vi "Channel Registration.vi"() -> ()   [LabVIEW 2021]
uses:
  Hardware Configuration/Hardware Configuration Controls/Device Type.ctl
  Hardware Configuration/Hardware Configuration Controls/Device Function.ctl
  <vilib>/vision/Image Controls.llb/IMAQ Image.ctl
  Channel Reg Controls/Channel Reg Notifier Type.ctl
  Channel Reg Controls/Channel Reg Actions.ctl
  Device Library/Cameras/Hamamatsu/Orca Flash/Orca Flash Controls/Orca Flash Actions.ctl
  Device Library/Stages/Stages Controls/Stage Actions.ctl
  Channel Reg Sub VI/Reg Counter Action.ctl
  Device Library/Cameras/Camera Controls/Camera IMAQ Key Info.ctl
  <vilib>/vision/NI_Vision_Development_Module.lvlib
panel:
  in  "Edge Size":i32
  in  "Base Save Path":path
  in  "Save Name":string
  in  "Subfolder Name":string="Area"
  in  "Quit":bool
  in  "No. of Steps":i32
  in  "Start Register":bool
  out "Bead Y Pos (µm)":dbl
  out "Bead X Pos (µm)":dbl
  in  "Move To Corner":bool
  in  "Pixel Size (µm)":dbl
  in  "Get Bead":bool
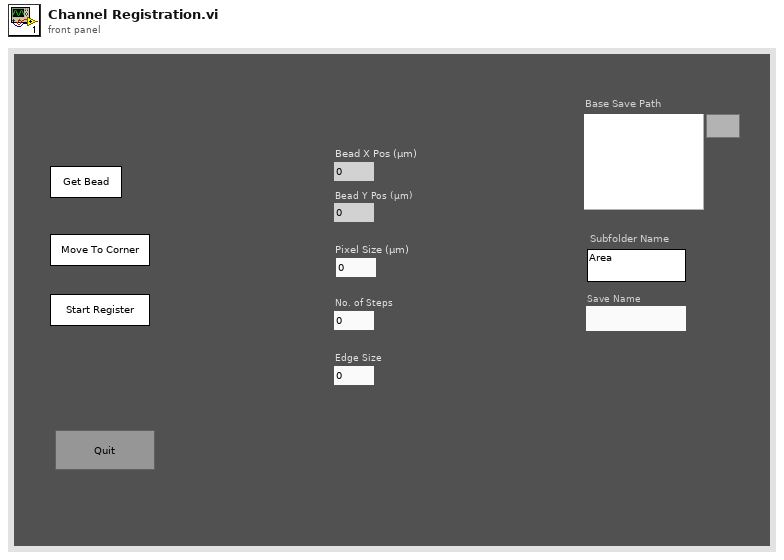
[diagram p1: front panel]
types:
  T1 = typedef "Orca Flash Actions.ctl" = enum16{"IDLE", "PREVIEW", "RECORD", "Send Trigger", "SOFT TRIGGER", "Record Settings", "SETPARAM", "GETPARAM", "SETROI", "GETROI", "PROGRESSIVE MODE", "AREA MODE", "STATUS", "QUIT"}
  T2 = typedef "Channel Reg Notifier Type.ctl" = cluster{"Action":T3, "Display Image":T4, "Init X Pos":dbl, "Init Y Pos":dbl, "Quads":T4[], "Add Quads":T4[], "Camera Image":T4, "Camera Notifier Name":string, "Stage Notifier Name":string, "X Grid Pos":dbl[], "Y Grid Pos":dbl[], "Pixel Size":dbl, "No. of Steps":i32, "Edge Size":i32, "Relative X":dbl, "Relative Y":dbl, "Scan Done?":bool}
  T3 = typedef "Channel Reg Actions.ctl" = enum16{"Start Register", "Get Bead", "Move To Corner", "Get Quad", "Add Quad", "Move Stage", "Save Image", "Exit", "Quit"}
  T4 = typedef "IMAQ Image.ctl" = refnum<image>
  T5 = typedef "Device Function.ctl" = enum16{"Primary", "Secondary", "Overview", "Wide Field Drift Correction", "642 nm Excitation", "560 nm Excitation", "940 nm Excitation", "546 nm Excitation", "488 nm Excitation", "405 nm Excitation", "Objective Drift Correction", "4Pi Focus Lock", "4Pi Objective Lock", "Objective XY", "Objective Z", "Sample XY", "Sample Coarse Z", "Sample Z", "4Pi Lower", "4Pi Upper", "Em Small", "Em Large", "Ex Small", "Ex Large", "Mojo", "Adj Cavity", "Line Scanning", "Alert"}
  T6 = typedef "Device Type.ctl" = enum16{"AOTF", "Camera", "Deformable Mirror", "Laser", "Flip Mirror", "Shutter", "Stage", "Waveform", "FPGA", "Email"}
  T7 = typedef "Image Type" = u32
  T8 = typedef "Stage Actions.ctl" = enum16{"Get Position", "SERVO OFF", "SERVO ON", "SERVO ON/OFF", "MVR", "MOVE", "HALT", "ONTARGET", "ERROR", "REFERENCE", "INIT", "VELOCITY", "STATUS", "EXIT", "HOME", "ZEROPOS", "NANOPOS", "ANALOG", "QUIT"}
  T9 = typedef "Reg Counter Action.ctl" = enum16{"Initialize", "Update Count"}
  T10 = typedef "Camera IMAQ Key Info.ctl" = cluster{"Frame":u32, "Sensor Height":i32, "Sensor Width":i32, "ROI Height":i32, "ROI Width":i32, "ROI Enable?":bool, "Bit per Pixel":u8}
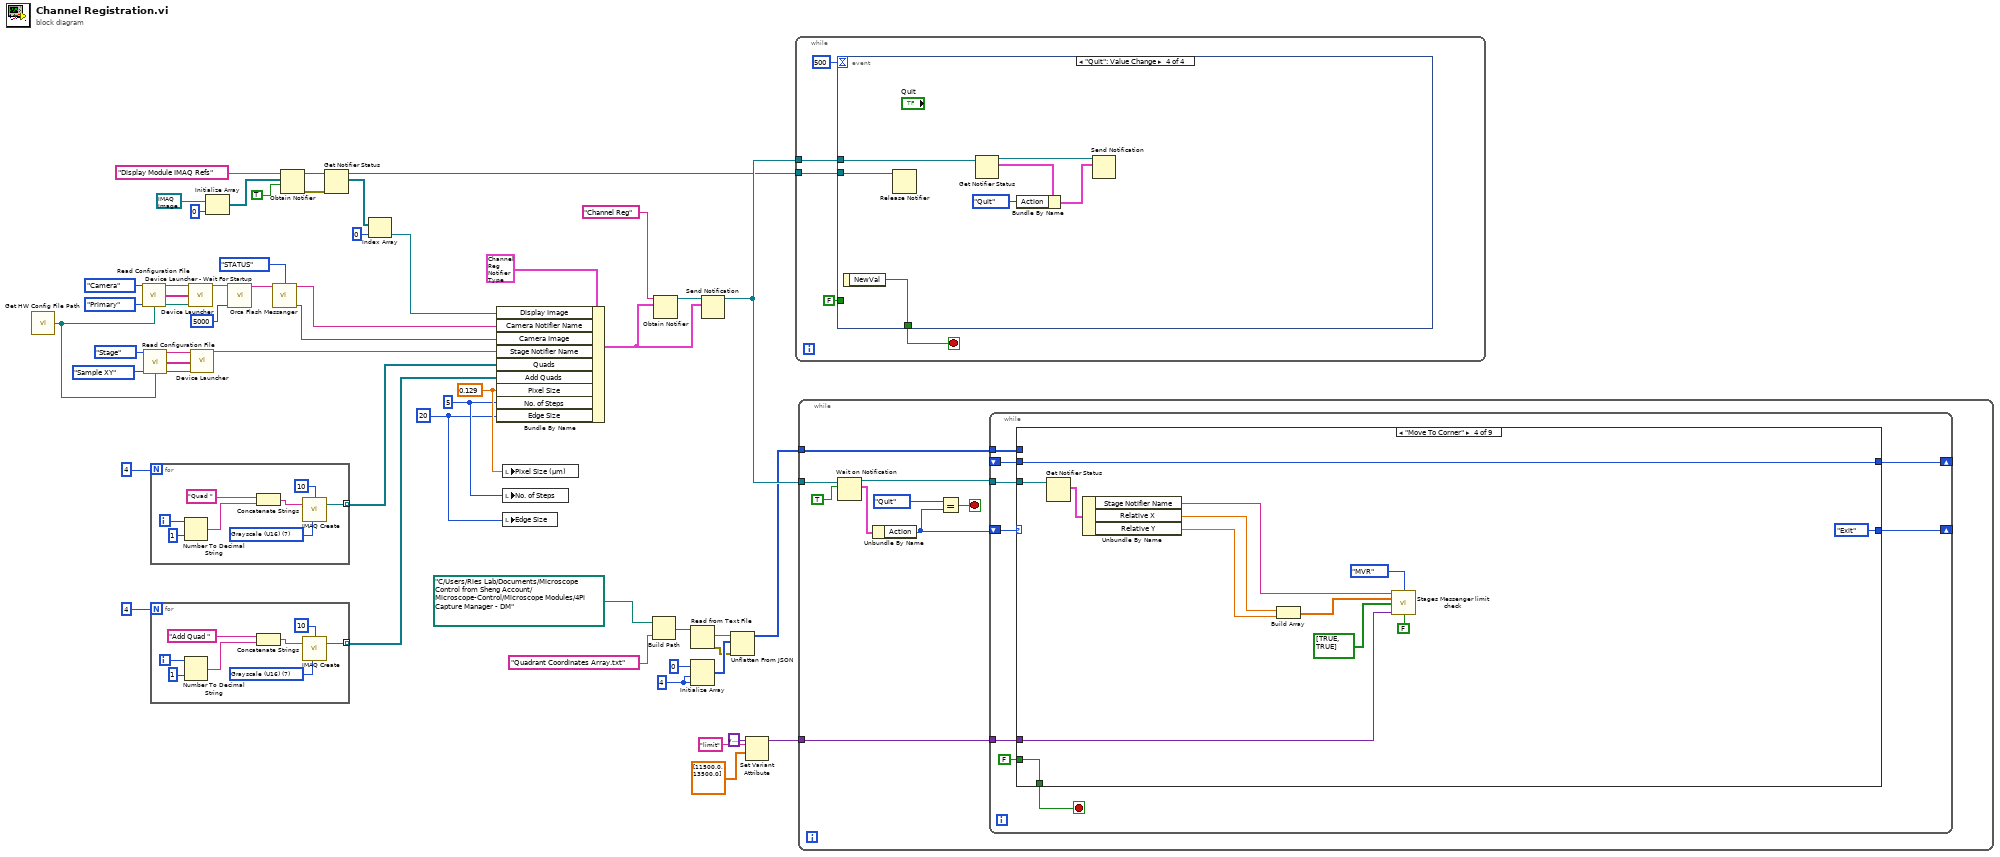
[diagram p0: block diagram]
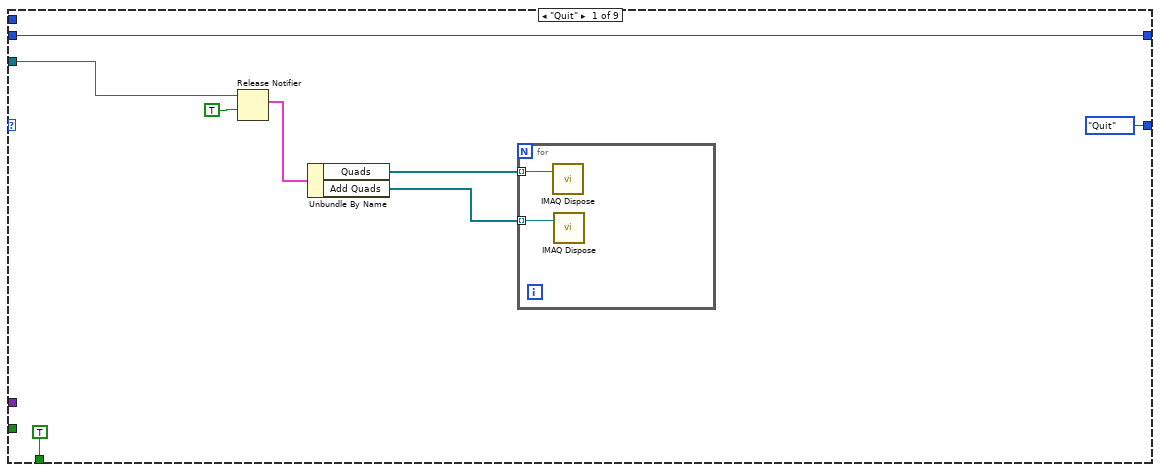
[diagram p2: hidden frame]
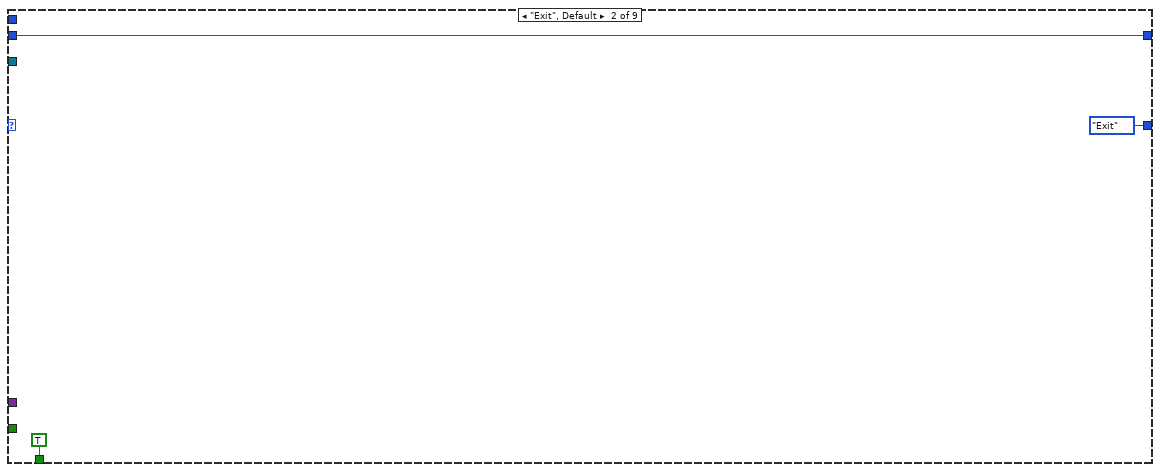
[diagram p3: hidden frame]
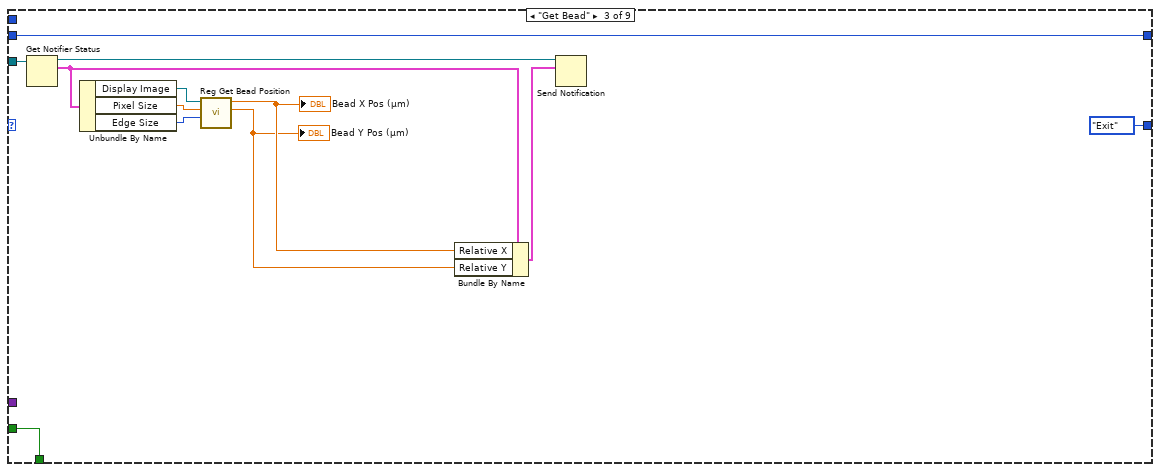
[diagram p4: hidden frame]
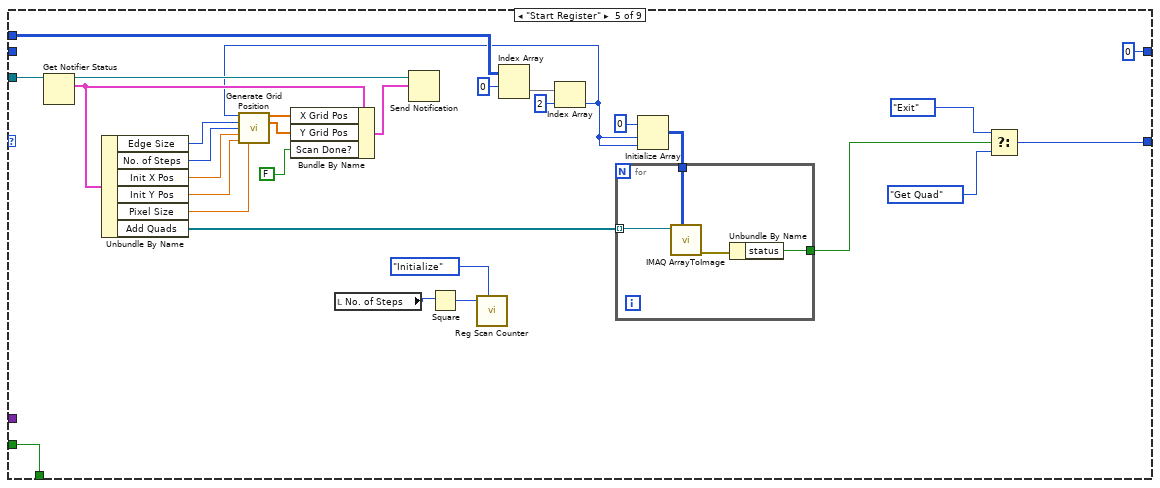
[diagram p5: hidden frame]
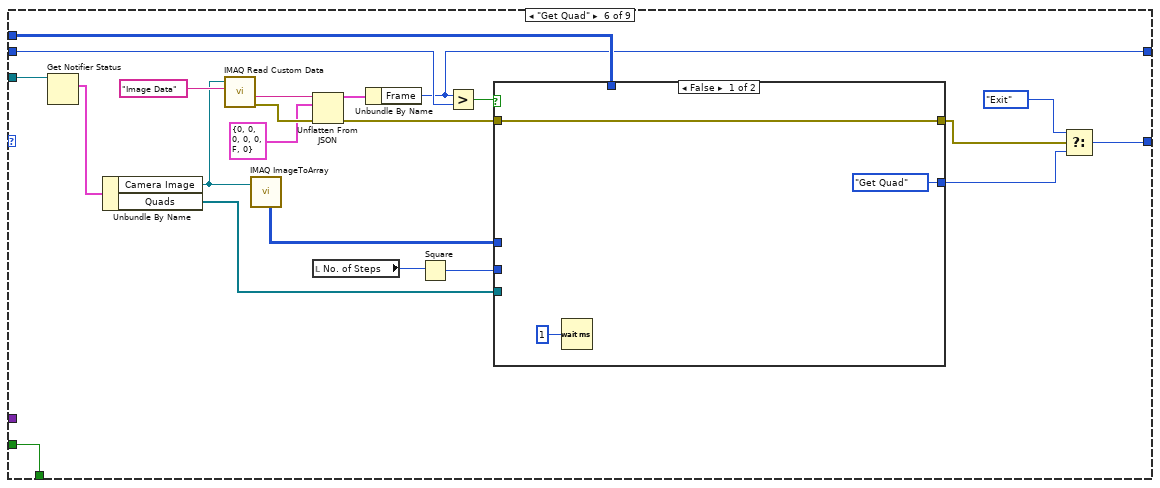
[diagram p6: hidden frame]
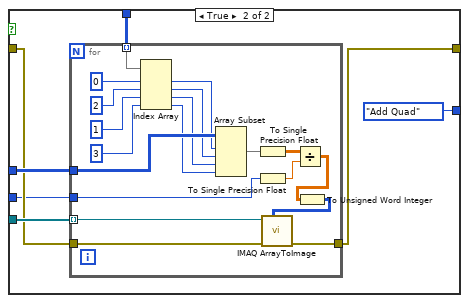
[diagram p7: hidden frame]
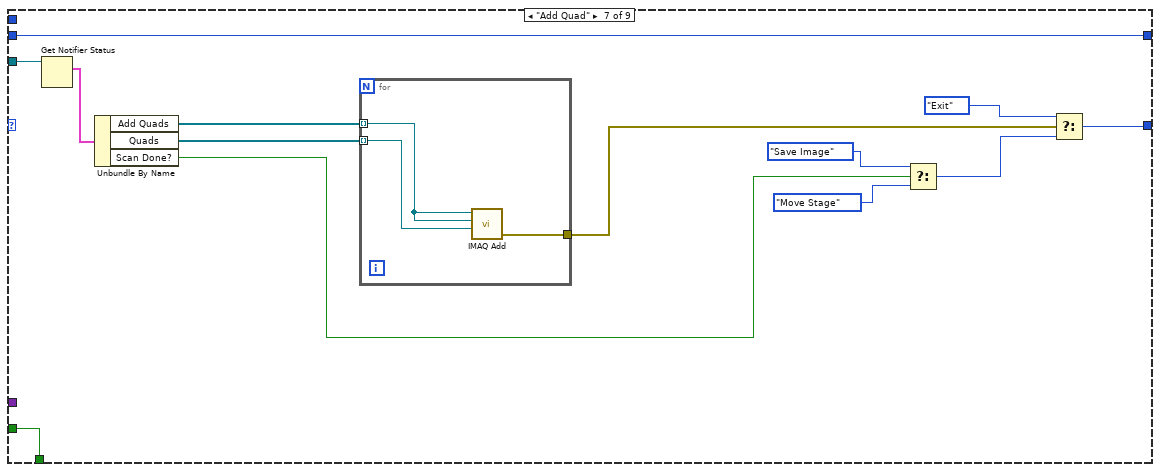
[diagram p8: hidden frame]
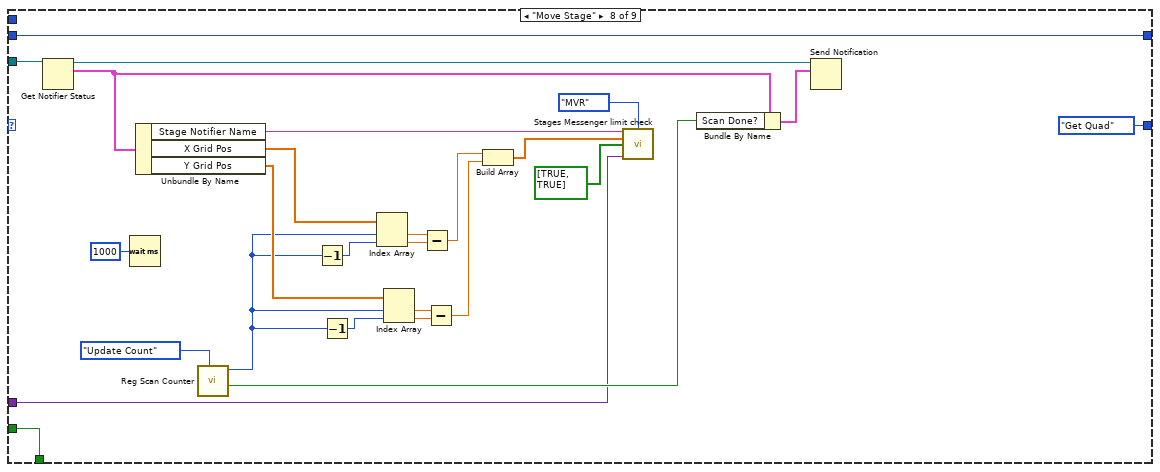
[diagram p9: hidden frame]
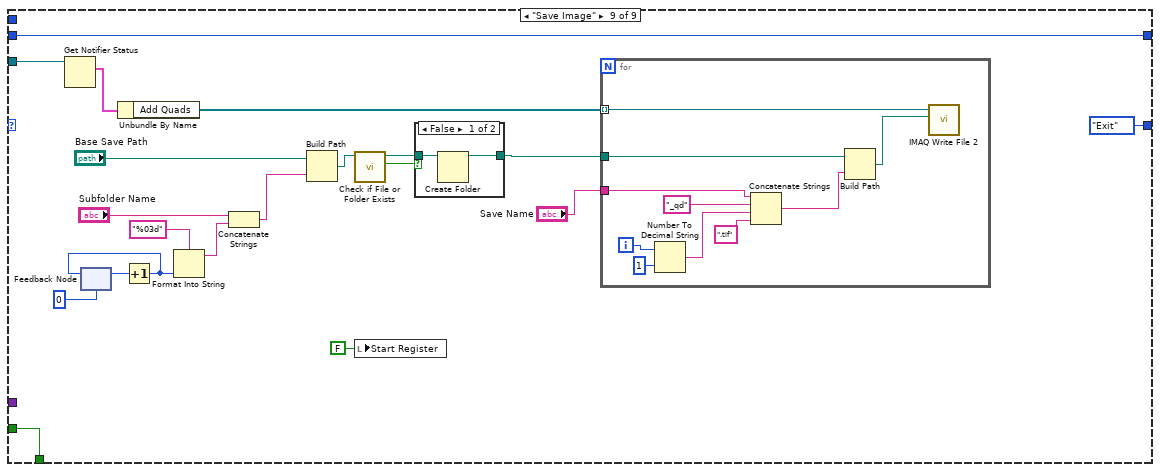
[diagram p10: hidden frame]
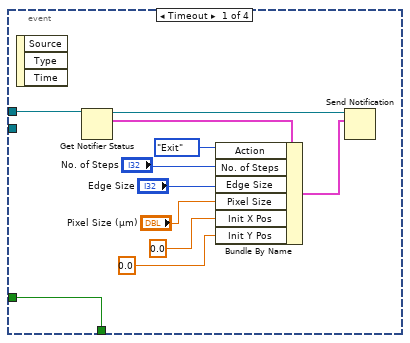
[diagram p12: hidden frame]
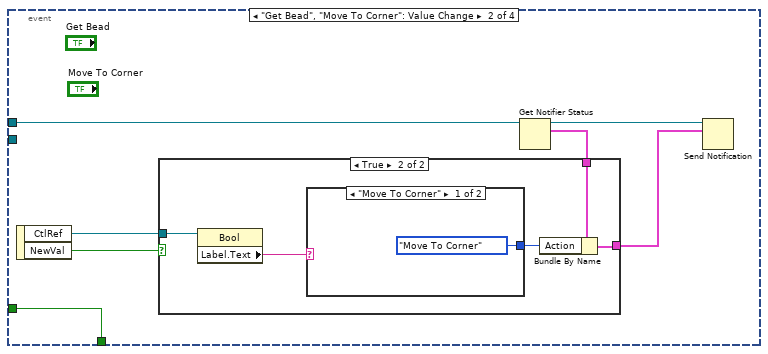
[diagram p13: hidden frame]
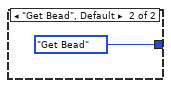
[diagram p15: hidden frame]
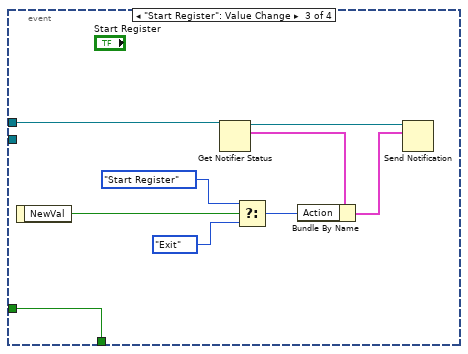
[diagram p16: hidden frame]
diagram:
  w1 = 20 ("Edge Size")
  w2 = 5 ("No. of Steps")
  w3 = 0.129 ("Pixel Size")
  w18 = 4 ("dimension size")
  n1 = call "Get HW Config File Path.vi"() -> ("File Path"=w49:path)  [unwired: 14 in, 1 out]
  n2 = call "Read Configuration File.vi"("Device Type"=Device_Type."Camera", "Device Function"=Device_Function."Primary", "Config File Path"=w49) -> ("Unique Notifier Name"=w50:string, "Device Ports/IDs/Channels"=w52:string[], "Device Engine Path"=w51:path)  [unwired: 9 in, 1 out]
  n3 = call "Read Configuration File.vi"("Device Type"=Device_Type."Stage", "Device Function"=Device_Function."Sample XY", "Config File Path"=w49) -> ("Unique Notifier Name"=w46:string, "Device Ports/IDs/Channels"=w45:string[], "Device Engine Path"=w44:path)  [unwired: 9 in, 1 out]
  n4 = for {
    N: 4 -> [_]
    tunnel: [w60] -> w27 mode=indexing
    i -> [w59]
    w62 = T7 7 items=["Grayscale (U8)", "Grayscale (I16)", "Grayscale (SGL)", "Complex (CSG)", "RGB (U32)", "HSL (U32)", "RGB (U64)", "Grayscale (U16)"] ("Image Type")
    n5 = Number To Decimal String(number=w59, width (-)=i16 1) -> (decimal integer string=w56:string)
    n6 = Concatenate Strings("Quad " ("Image Name"), w56) -> (w55:string)
    n7 = call "IMAQ Create"("Border Size"=10, "Image Name"=w55, "Image Type"=w62) -> ("New Image"=w60:T4)  [unwired: 2 in, 1 out]
  }
  n8 = for {
    N: 4 -> [_]
    tunnel: [w68] -> w25 mode=indexing
    i -> [w67]
    w70 = T7 7 items=["Grayscale (U8)", "Grayscale (I16)", "Grayscale (SGL)", "Complex (CSG)", "RGB (U32)", "HSL (U32)", "RGB (U64)", "Grayscale (U16)"] ("Image Type")
    n9 = Number To Decimal String(number=w67, width (-)=i16 1) -> (decimal integer string=w64:string)
    n10 = Concatenate Strings("Add Quad " ("Image Name"), w64) -> (w63:string)
    n11 = call "IMAQ Create"("Border Size"=10, "Image Name"=w63, "Image Type"=w70) -> ("New Image"=w68:T4)  [unwired: 2 in, 1 out]
  }
  n12 = call "Device Launcher.vi"("Notifier Name"=w50, "Device Ports/IDs/Channels"=w52, "Device Engine Path"=w51) -> ("Notifier Name"=w16:string)  [unwired: 11 in, 1 out]
  n13 = call "Device Launcher.vi"("Notifier Name"=w46, "Device Ports/IDs/Channels"=w45, "Device Engine Path"=w44) -> ("Notifier Name"=w10:string)  [unwired: 11 in, 1 out]
  n14 = Initialize Array(T4 refnum ("New Image"), 0 ("dimension size")) -> (w39:T4[])
  n15 = call "Device Launcher - Wait For Startup.vi"("Notifier Name"=w16, "Wait Time (ms)"=5000) -> ("Notifier Name (Dup)"=w14:string)  [unwired: 12 in, 1 out]
  n16 = call "Orca Flash Messanger.vi"("Notifier Name"=w14, "Camera Actions"=Orca_Flash_Actions."STATUS") -> ("Notifier Name Dup"=w11:string, "Image Ref"=w12:T4)  [unwired: 9 in, 3 out]
  n17 = Obtain Notifier(name (unnamed)="Display Module IMAQ Refs", notification data type=w39, create if not found? (T)=TRUE) -> (notifier out=w38:refnum<notifier>, error out=w37:errorcluster)  [unwired: 1 in, 1 out]
  n18 = Get Notifier Status(notifier=w38, error in (no error)=w37) -> (notifier out=w9:refnum<notifier>, current notification=w36:T4[])  [unwired: 3 out]
  n19 = Index Array(array=w36, index=0) -> (element=w33:T4)
  n20 = Bundle By Name(cluster=T2 {"Action"=enum."Get Bead", "Display Image"=refnum, "Init X Pos"=0.0, "Init Y Pos"=0.0, "Quads"=[], "Add Quads"=[], "Camera Image"=refnum, "Camera Notifier Name"="", "Stage Notifier Name"="", "X Grid Pos"=[], "Y Grid Pos"=[], "Pixel Size"=0.0, "No. of Steps"=0, "Edge Size"=0, "Relative X"=0.0, "Relative Y"=0.0, "Scan Done?"=FALSE} ("Channel Reg Notifier Type"), "Display Image"=w33, "Camera Notifier Name"=w11, "Camera Image"=w12, "Stage Notifier Name"=w10, "Quads"=w27, "Add Quads"=w25, "Pixel Size"=w3, "No. of Steps"=w2, "Edge Size"=w1) -> (w30:T2)
  n21 = local write "Pixel Size (µm)"(w3) -> ()
  n22 = local write "No. of Steps"(w2) -> ()
  n23 = local write "Edge Size"(w1) -> ()
  n24 = Build Path(base path=path "C:/Users/Ries Lab/Documents/Microscope Control from Sheng Account/Microscope-Control/Microscope Modules/4Pi Capture Manager - DM" ("path"), name or relative path="Quadrant Coordinates Array.txt") -> (appended path=w21:path)
  n25 = Obtain Notifier(name (unnamed)="Channel Reg", notification data type=w30) -> (notifier out=w31:refnum<notifier>)  [unwired: 2 in, 2 out]
  n26 = Read from Text File(file (use dialog)=w21) -> (text=w20:string, error out=w19:errorcluster)  [unwired: 3 in, 2 out]
  n27 = Initialize Array(0 ("element"), w18, w18) -> (w22:i32[][])
  n28 = Send Notification(notification=w30, notifier=w31) -> (notifier out=w29:refnum<notifier>)  [unwired: 1 in, 1 out]
  n29 = Unflatten From JSON(JSON string=w20, type and defaults=w22, error in (no error)=w19) -> (value=w17:i32[][])  [unwired: 4 in, 1 out]
  n30 = Set Variant Attribute(Variant=variant ("variant"), name="limit", value=dbl[] [11500.0, 13500.0] ("Array")) -> (Variant out=w5:variant)  [unwired: 1 in, 2 out]
  n31 = while {
    tunnel: w29 -> [w75]
    tunnel: w9 -> [w72]
    stop <- w74 stop-if-true
    n32 = event shown="[3] \"Quit\": Value Change" {
      selector: _ -> [_ _ _ _]
      dyn-events: _ -> [_ _ _ _]
      timeout: 500 -> [_ _ _ _]
      tunnel: w75 -> [w85 w93 w110 w116]
      tunnel: [w86 w87 w102 w117] -> w74
      tunnel: FALSE ("NewVal") -> [w86 w87 w102 _]
      tunnel: w72 -> [_ _ _ w111]
      event Timeout {
        n33 = event-data() -> ()  [unwired: 1 in, 3 out]
        n34 = Get Notifier Status(notifier=w85) -> (notifier out=w78:refnum<notifier>, current notification=w84:T2)  [unwired: 1 in, 3 out]
        n35 = Bundle By Name(cluster=w84, "Action"=Channel_Reg_Actions."Exit", "No. of Steps"="No. of Steps", "Edge Size"="Edge Size", "Pixel Size"="Pixel Size (µm)", "Init X Pos"=0.0, "Init Y Pos"=0.0) -> (w77:T2)
        n36 = Send Notification(notification=w77, notifier=w78) -> ()  [unwired: 1 in, 2 out]
      }
      event "Get Bead", "Move To Corner": Value Change {
        n37 = event-data() -> ("CtlRef"=w88:refnum<vi>, "NewVal"=w89:bool)  [unwired: 1 in]
        n38 = Get Notifier Status(notifier=w93) -> (notifier out=w91:refnum<notifier>, current notification=w92:T2)  [unwired: 1 in, 3 out]
        n39 = case shown="True" w89 {
          tunnel: w92 -> [w94 w99]
          tunnel: [w94 w97] -> w90
          tunnel: w88 -> [_ w96]
          frame False {
          }
          frame True {
            n40 = property class="Bool"(reference=w96) -> ("Label.Text"=w95:string)  [unwired: 1 in, 2 out]
            n41 = case shown="\"Move To Corner\"" w95 {
              tunnel: [Channel_Reg_Actions."Move To Corner" ("Action") Channel_Reg_Actions."Get Bead" ("Action")] -> w98
              frame "Move To Corner" {
              }
              frame "Get Bead", Default {
              }
            }
            n42 = Bundle By Name(cluster=w99, "Action"=w98) -> (w97:T2)
          }
        }
        n43 = Send Notification(notification=w90, notifier=w91) -> ()  [unwired: 1 in, 2 out]
      }
      event "Start Register": Value Change {
        n44 = event-data() -> ("NewVal"=w108:bool)  [unwired: 1 in]
        n45 = Get Notifier Status(notifier=w110) -> (notifier out=w104:refnum<notifier>, current notification=w109:T2)  [unwired: 1 in, 3 out]
        n46 = Select(t=Channel_Reg_Actions."Start Register" ("x"), s=w108, f=Channel_Reg_Actions."Exit") -> (s? t:f=w105:T3)
        n47 = Bundle By Name(cluster=w109, "Action"=w105) -> (w103:T2)
        n48 = Send Notification(notification=w103, notifier=w104) -> ()  [unwired: 1 in, 2 out]
      }
      event "Quit": Value Change {
        n49 = event-data() -> ("NewVal"=w117:bool)  [unwired: 1 in]
        n50 = Release Notifier(notifier=w111) -> ()  [unwired: 2 in, 3 out]
        n51 = Get Notifier Status(notifier=w116) -> (notifier out=w115:refnum<notifier>, current notification=w114:T2)  [unwired: 1 in, 3 out]
        n52 = Bundle By Name(cluster=w114, "Action"=Channel_Reg_Actions."Quit") -> (w113:T2)
        n53 = Send Notification(notification=w113, notifier=w115) -> ()  [unwired: 1 in, 2 out]
      }
    }
  }
  n54 = while {
    tunnel: w29 -> [w126]
    tunnel: w17 -> [w119]
    tunnel: w5 -> [w118]
    stop <- w120 stop-if-true
    n55 = Wait on Notification(notifier=w126, ignore previous (F)=TRUE) -> (notifier out=w123:refnum<notifier>, notification=w124:T2)  [unwired: 2 in, 2 out]
    n56 = Unbundle By Name(w124) -> ("Action"=w122:T3)
    n57 = Equal?(x=Channel_Reg_Actions."Quit", y=w122) -> (x = y?=w120:bool)
    n58 = while {
      tunnel: w123 -> [w135]
      tunnel: w119 -> [w133]
      shift-right: [w132] -> _
      shift-left: w122 -> [w134]
      shift-right: [w130] -> _
      shift-left: _ -> [w131]
      tunnel: w118 -> [w127]
      stop <- w129 stop-if-true
      n59 = case shown="\"Move To Corner\"" w134 {
        tunnel: w135 -> [w143 _ w160 w169 w202 w228 w270 w299 w319]
        tunnel: w133 -> [_ _ _ _ w198 w219 _ _ _]
        tunnel: [Channel_Reg_Actions."Quit" ("f") Channel_Reg_Actions."Exit" ("f") Channel_Reg_Actions."Exit" ("f") Channel_Reg_Actions."Exit" ("f") w191 w212 w263 Channel_Reg_Actions."Get Quad" ("f") Channel_Reg_Actions."Exit" ("f")] -> w132
        tunnel: w131 -> [w142 w148 w155 w167 _ w221 w269 w293 w303]
        tunnel: [w142 w148 w155 w167 u32 0 ("Frame") w210 w269 w293 w303] -> w130
        tunnel: [TRUE TRUE w153 w165 w186 w209 w262 w292 w301] -> w129
        tunnel: FALSE -> [_ _ w153 w165 w186 w209 w262 w292 w301]
        tunnel: w127 -> [_ _ _ w161 _ _ _ w274 _]
        frame "Quit" {
          n60 = Release Notifier(notifier=w143, force destroy? (F)=TRUE) -> (last notification=w140:T2)  [unwired: 1 in, 2 out]
          n61 = Unbundle By Name(w140) -> ("Quads"=w137:T4[], "Add Quads"=w136:T4[])
          n62 = for {
            tunnel: w137 -> [w145] mode=indexing
            tunnel: w136 -> [w144] mode=indexing
            n63 = call "IMAQ Dispose"("Image"=w145) -> ()  [unwired: 5 in, 1 out]
            n64 = call "IMAQ Dispose"("Image"=w144) -> ()  [unwired: 5 in, 1 out]
          }
        }
        frame "Exit", Default {
        }
        frame "Get Bead" {
          n65 = Get Notifier Status(notifier=w160) -> (notifier out=w158:refnum<notifier>, current notification=w157:T2)  [unwired: 1 in, 3 out]
          n66 = Unbundle By Name(w157) -> ("Display Image"=w159:T4, "Pixel Size"=w150:dbl, "Edge Size"=w149:i32)
          n67 = call "Reg Get Bead Position.vi"("Edge size"=w149, "Pixel Size (µm)"=w150, "Image Ref"=w159) -> ("Y Pos"=w151:dbl, "X Pos"=w152:dbl)  [unwired: 7 in]
          "Bead X Pos (µm)" <- w152
          "Bead Y Pos (µm)" <- w151
          n68 = Bundle By Name(cluster=w157, "Relative X"=w152, "Relative Y"=w151) -> (w156:T2)
          n69 = Send Notification(notification=w156, notifier=w158) -> ()  [unwired: 1 in, 2 out]
        }
        frame "Move To Corner" {
          n70 = Get Notifier Status(notifier=w169) -> (current notification=w162:T2)  [unwired: 1 in, 4 out]
          n71 = Unbundle By Name(w162) -> ("Stage Notifier Name"=w168:string, "Relative X"=w163:dbl, "Relative Y"=w164:dbl)
          n72 = Build Array(w163, w164) -> (w171:dbl[])
          n73 = call "Stages Messenger limit check.vi"("Stage Notifier Name"=w168, "Actions"=Stage_Actions."MVR", "Setpoint"=w171, "Axis"=bool[] [TRUE, TRUE], "Misc"=w161, "Exit While Busy?"=FALSE) -> ()  [unwired: 6 in, 4 out]
        }
        frame "Start Register" {
          n74 = Get Notifier Status(notifier=w202) -> (notifier out=w185:refnum<notifier>, current notification=w188:T2)  [unwired: 1 in, 3 out]
          n75 = Unbundle By Name(w188) -> ("Edge Size"=w182:i32, "No. of Steps"=w183:i32, "Init X Pos"=w178:dbl, "Init Y Pos"=w177:dbl, "Pixel Size"=w184:dbl, "Add Quads"=w195:T4[])
          n76 = local read "No. of Steps"() -> (w175:i32)
          n77 = Square(x=w175) -> (x^2=w176:i32)
          n78 = call "Reg Scan Counter.vi"("Action"=Reg_Counter_Action."Initialize", "# of Steps"=w176) -> ()  [unwired: 8 in, 2 out]
          n79 = Index Array(array=w198, index (row)=0) -> (element=w200:i32[])  [unwired: 1 in]
          n80 = Index Array(array=w200, index=2) -> (element=w181:i32)
          n81 = call "Generate Grid Position.vi"("Image Size"=w181, "Edge Size"=w182, "# of Steps"=w183, "init x pos"=w178, "init y pos"=w177, "Pixel Size"=w184) -> ("x grid pos"=w180:dbl[], "y grid pos"=w179:dbl[])  [unwired: 8 in]
          n82 = Bundle By Name(cluster=w188, "X Grid Pos"=w180, "Y Grid Pos"=w179, "Scan Done?"=FALSE) -> (w187:T2)
          n83 = Send Notification(notification=w187, notifier=w185) -> ()  [unwired: 1 in, 2 out]
          n84 = Initialize Array(u16 0 ("index"), w181, w181) -> (w196:u16[][])
          n85 = for {
            tunnel: w196 -> [w206]
            tunnel: w195 -> [w205] mode=indexing
            tunnel: [w203] -> w194
            n86 = call "IMAQ ArrayToImage"("Image Pixels (U16)"=w206, "Image"=w205) -> ("error out"=w204:errorcluster)  [unwired: 8 in, 1 out]
            n87 = Unbundle By Name(w204) -> ("status"=w203:bool)
          }
          n88 = Select(t=Channel_Reg_Actions."Exit" ("x"), s=w194, f=Channel_Reg_Actions."Get Quad") -> (s? t:f=w191:T3)
        }
        frame "Get Quad" {
          n89 = Get Notifier Status(notifier=w228) -> (current notification=w227:T2)  [unwired: 1 in, 4 out]
          n90 = Unbundle By Name(w227) -> ("Camera Image"=w218:T4, "Quads"=w216:T4[])
          n91 = call "IMAQ Read Custom Data"("Key"="Image Data", "Image"=w218) -> ("error out"=w226:errorcluster, "Custom Data Out"=w225:string)  [unwired: 7 in, 1 out]
          n92 = call "IMAQ ImageToArray"("Image"=w218) -> ("Image Pixels (U16)"=w217:u16[][])  [unwired: 3 in, 4 out]
          n93 = Unflatten From JSON(JSON string=w225, type and defaults=T10 {"Frame"=0, "Sensor Height"=0, "Sensor Width"=0, "ROI Height"=0, "ROI Width"=0, "ROI Enable?"=FALSE, "Bit per Pixel"=0} ("Camera IMAQ Key Info"), error in (no error)=w226) -> (value=w223:T10, error out=w215:errorcluster)  [unwired: 4 in]
          n94 = local read "No. of Steps"() -> (w208:i32)
          n95 = Unbundle By Name(w223) -> ("Frame"=w210:u32)
          n96 = Square(x=w208) -> (x^2=w207:i32)
          n97 = Greater?(x=w210, y=w221) -> (0:w220:bool)
          n98 = case shown="False" w220 {
            tunnel: w216 -> [_ w238]
            tunnel: w219 -> [_ w237]
            tunnel: w217 -> [_ w236]
            tunnel: w215 -> [w230 w235]
            tunnel: [w230 w234] -> w214
            tunnel: [Channel_Reg_Actions."Get Quad" ("f") Channel_Reg_Actions."Add Quad" ("f")] -> w211
            tunnel: w207 -> [_ w232]
            frame False {
              n99 = Wait (ms)(milliseconds to wait=u32 1) -> ()  [unwired: 1 out]
            }
            frame True {
              n100 = for {
                tunnel: w238 -> [w256] mode=indexing
                tunnel: w236 -> [w257]
                tunnel: w237 -> [w255] mode=indexing
                tunnel: [w246] -> w234
                tunnel: w235 -> [w245]
                tunnel: w232 -> [w242]
                n101 = Index Array(array=w255, index #1=0 ("index"), index #2=2 ("index"), index #3=1 ("index"), index #4=3 ("index")) -> (element #1=w253:i32, element #2=w252:i32, element #3=w248:i32, element #4=w247:i32)
                n102 = Array Subset(array=w257, index (row)=w253, length (row)=w252, index (col)=w248, length (col)=w247) -> (w244:u16[][])
                n103 = To Single Precision Float(number=w244) -> (single precision float=w243:sgl[][])
                n104 = To Single Precision Float(number=w242) -> (single precision float=w241:sgl)
                n105 = Divide(x=w243, y=w241) -> (x/y=w240:sgl[][])
                n106 = To Unsigned Word Integer(number=w240) -> (unsigned 16bit integer=w239:u16[][])
                n107 = call "IMAQ ArrayToImage"("Image Pixels (U16)"=w239, "error in (no error)"=w245, "Image"=w256) -> ("error out"=w246:errorcluster)  [unwired: 7 in, 1 out]
              }
            }
          }
          n108 = Select(t=Channel_Reg_Actions."Exit" ("x"), s=w214, f=w211) -> (s? t:f=w212:T3)
        }
        frame "Add Quad" {
          n109 = Get Notifier Status(notifier=w270) -> (current notification=w268:T2)  [unwired: 1 in, 4 out]
          n110 = Unbundle By Name(w268) -> ("Add Quads"=w266:T4[], "Quads"=w267:T4[], "Scan Done?"=w260:bool)
          n111 = for {
            tunnel: w267 -> [w273] mode=indexing
            tunnel: w266 -> [w271] mode=indexing
            tunnel: [w272] -> w265
            n112 = call "IMAQ Add"("Image Src A"=w271, "Image Dst"=w271, "Image Src B"=w273) -> ("error out"=w272:errorcluster)  [unwired: 4 in, 1 out]
          }
          n113 = Select(t=Channel_Reg_Actions."Save Image", s=w260, f=Channel_Reg_Actions."Move Stage") -> (s? t:f=w258:T3)
          n114 = Select(t=Channel_Reg_Actions."Exit" ("x"), s=w265, f=w258) -> (s? t:f=w263:T3)
        }
        frame "Move Stage" {
          n115 = Get Notifier Status(notifier=w299) -> (notifier out=w278:refnum<notifier>, current notification=w277:T2)  [unwired: 1 in, 3 out]
          n116 = Wait (ms)(milliseconds to wait=u32 1000) -> ()  [unwired: 1 out]
          n117 = Unbundle By Name(w277) -> ("Stage Notifier Name"=w297:string, "X Grid Pos"=w282:dbl[], "Y Grid Pos"=w298:dbl[])
          n118 = call "Reg Scan Counter.vi"("Action"=Reg_Counter_Action."Update Count") -> ("Scan Done?"=w276:bool, "Current Step"=w290:i32)  [unwired: 9 in]
          n119 = Decrement(x=w290) -> (x-1=w291:i32)
          n120 = Decrement(x=w290) -> (x-1=w289:i32)
          n121 = Index Array(array=w282, index #1=w290, index #2=w291) -> (element #1=w281:dbl, element #2=w288:dbl)
          n122 = Index Array(array=w298, index #1=w290, index #2=w289) -> (element #1=w280:dbl, element #2=w286:dbl)
          n123 = Subtract(x=w281, y=w288) -> (x-y=w287:dbl)
          n124 = Subtract(x=w280, y=w286) -> (x-y=w285:dbl)
          n125 = Build Array(w287, w285) -> (w284:dbl[])
          n126 = call "Stages Messenger limit check.vi"("Stage Notifier Name"=w297, "Actions"=Stage_Actions."MVR", "Setpoint"=w284, "Axis"=bool[] [TRUE, TRUE], "Misc"=w274) -> ()  [unwired: 7 in, 4 out]
          n127 = Bundle By Name(cluster=w277, "Scan Done?"=w276) -> (w275:T2)
          n128 = Send Notification(notification=w275, notifier=w278) -> ()  [unwired: 1 in, 2 out]
        }
        frame "Save Image" {
          n129 = Get Notifier Status(notifier=w319) -> (current notification=w318:T2)  [unwired: 1 in, 4 out]
          n130 = feedback #1(u32 0) -> (w312:u32)
          n131 = Unbundle By Name(w318) -> ("Add Quads"=w317:T4[])
          n132 = Increment(x=w312) -> (x+1=w311:u32)
          n133 = feedback-in #1(w311) -> ()
          n134 = Format Into String(format string="%03d", w311) -> (resulting string=w313:string)  [unwired: 2 in, 1 out]
          n135 = Concatenate Strings("Subfolder Name", w313) -> (w310:string)
          n136 = Build Path(base path="Base Save Path", name or relative path=w310) -> (appended path=w307:path)
          n137 = call <vilib>:"Check if File or Folder Exists.vi"("path"=w307) -> ("file or folder exists?"=w309:bool, "dup path"=w308:path)  [unwired: 8 in, 1 out]
          n138 = local write "Start Register"(FALSE ("Start Register")) -> ()
          n139 = case shown="False" w309 {
            tunnel: [w320 w322] -> w306
            tunnel: w308 -> [w321 w322]
            frame False {
              n140 = Create Folder(path (use dialog)=w321) -> (created path=w320:path)  [unwired: 2 in, 2 out]
            }
            frame True {
            }
          }
          n141 = for {
            tunnel: w317 -> [w332] mode=indexing
            tunnel: w306 -> [w331]
            tunnel: "Save Name" -> [w325]
            i -> [w327]
            n142 = Number To Decimal String(number=w327, width (-)=i16 1) -> (decimal integer string=w328:string)
            n143 = Concatenate Strings(w325, "_qd" ("Image Name"), w328, ".tif") -> (w324:string)
            n144 = Build Path(base path=w331, name or relative path=w324) -> (appended path=w323:path)
            n145 = call-poly "IMAQ Write File 2"("File Path"=w323, "Image"=w332) -> ()  [unwired: 8 in, 2 out]
          }
        }
      }
    }
  }
